vi "HS_DAQ_Host.vi"() -> ()   [LabVIEW 2020]
panel:
  out "Temperature [°C]":dbl format="%#_3g"
  out "Pulse count":dbl format="%#_3g"
  out "Frequency [Hz]":dbl format="%#_3g"
  out "Waveform Chart":dbl[][](graph)
  in  "Log data":bool
  in  "Sample rate [Hz]":dbl=20000.0
  in  "stop":bool
  out "data out":dbl[][](array[numeric]) format="%#_3g"
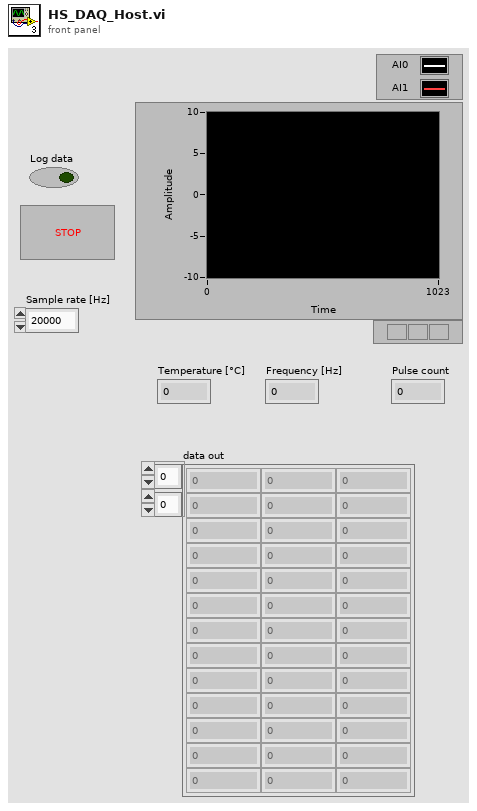
[diagram p1: front panel]
types:
  T1 = enum16{"open", "open or create", "create or replace", "create", "open (read-only)"}
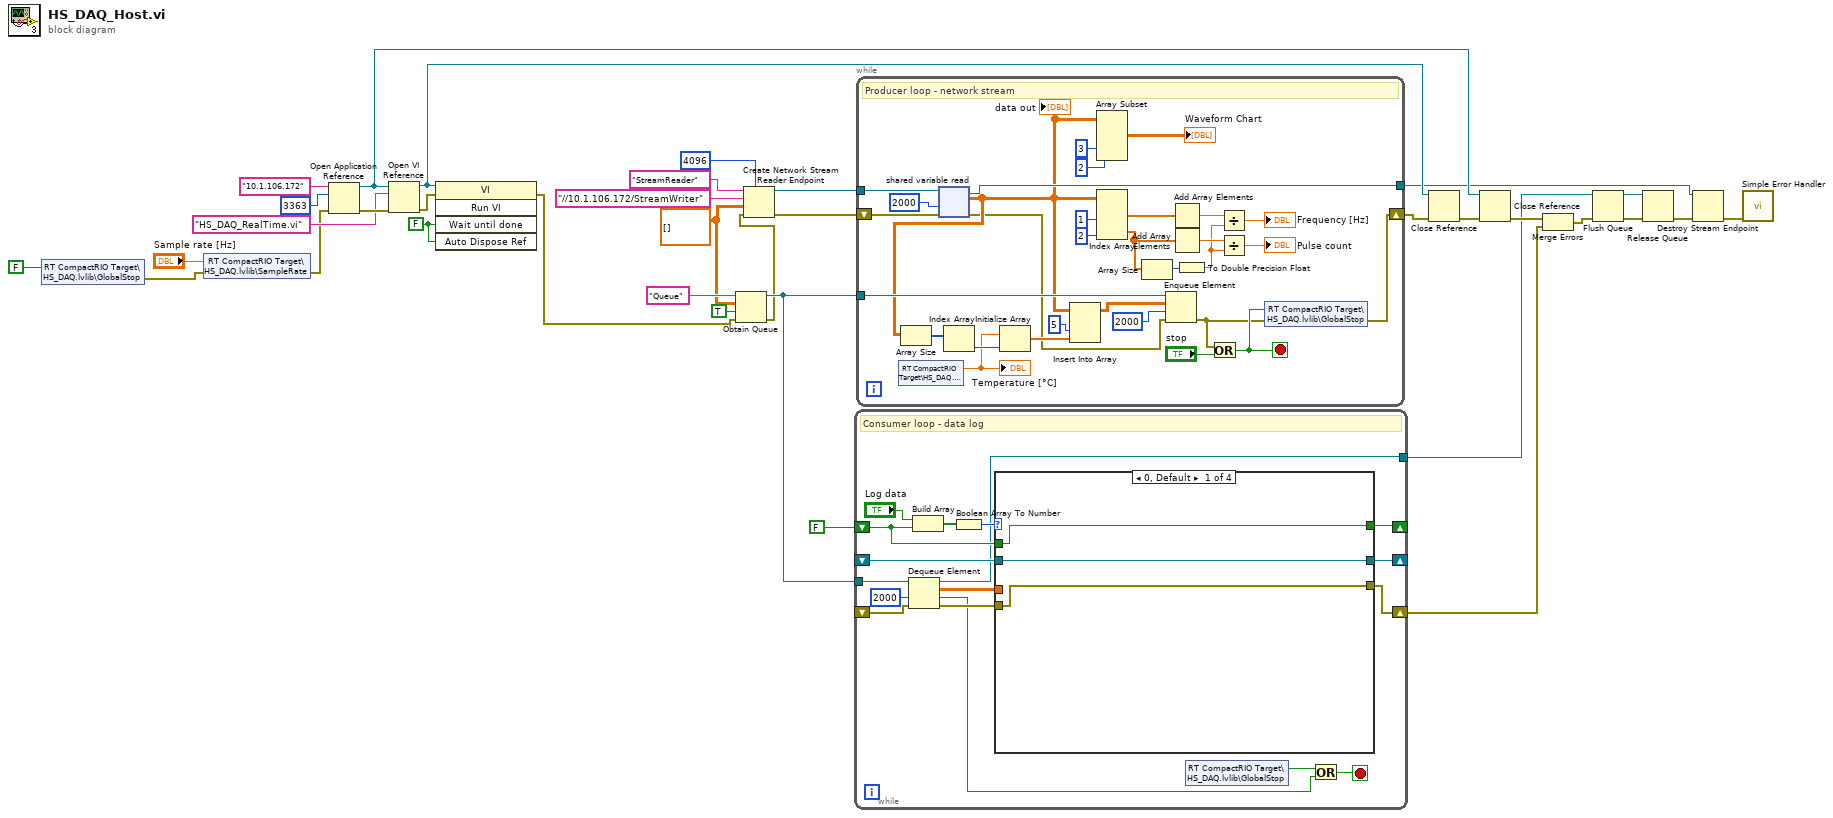
[diagram p0: block diagram]
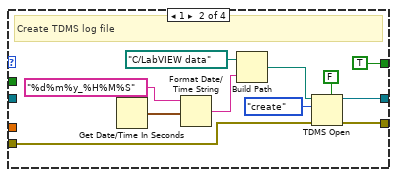
[diagram p2: hidden frame]
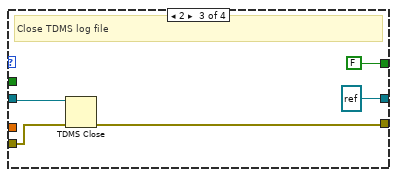
[diagram p3: hidden frame]
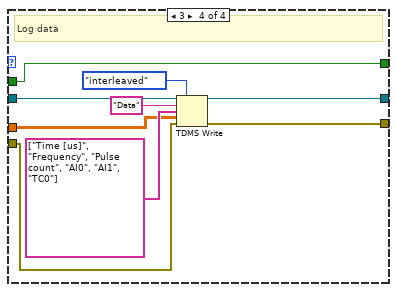
[diagram p4: hidden frame]
diagram:
  w26 = FALSE ("Wait Until Done")
  w24 = dbl[][] []
  n1 = shared-variable "RT CompactRIO Target\\HS_DAQ.lvlib\\GlobalStop"(FALSE ("GlobalStop")) -> (error out=w13:errorcluster)  [unwired: 1 in]
  n2 = shared-variable "RT CompactRIO Target\\HS_DAQ.lvlib\\SampleRate"("Sample rate [Hz]", error in=w13) -> (error out=w12:errorcluster)
  n3 = Open Application Reference(8:w12, 10:u16 3363 ("port number or service name (3363)"), 11:"10.1.106.172" ("machine name (\"\":  open local reference)")) -> (0:w29:errorcluster, 3:w19:refnum<vi>)  [unwired: 1 in]
  n4 = Open VI Reference(application reference (local)=w19, vi path="HS_DAQ_RealTime.vi" ("machine name (\"\":  open local reference)"), error in (no error)=w29) -> (vi reference=w20:refnum<vi>, error out=w27:errorcluster)  [unwired: 3 in]
  n5 = invoke class="VI" method="Run VI"(reference=w20, error in=w27, "Wait until done"=w26, "Auto Dispose Ref"=w26) -> (error out=w8:errorcluster)  [unwired: 1 in, 4 out]
  n6 = Obtain Queue(name (unnamed)="Queue", element data type=w24, create if not found? (T)=TRUE, error in (no error)=w8) -> (queue out=w23:refnum<queue>, error out=w7:errorcluster)  [unwired: 1 in, 1 out]
  n7 = Create Network Stream Reader Endpoint(7:4096 ("reader buffer size"), 8:w7, 9:w24, 10:"//10.1.106.172/StreamWriter" ("writer url"), 11:"StreamReader" ("reader name")) -> (0:w6:errorcluster, 3:w32:refnum<k21>)  [unwired: 2 in]
  n8 = while {
    tunnel: w23 -> [w52]
    shift-right: [w47] -> _
    shift-left: _ -> [w45]
    shift-right: [w46] -> _
    shift-left: FALSE -> [w44]
    shift-right: [w40] -> w3
    shift-left: _ -> [w42]
    tunnel: [w39] -> w1
    stop <- w38 stop-if-true
    # "Consumer loop - data log"
    n9 = Dequeue Element(queue=w52, timeout in ms (-1)=2000, error in (no error)=w42) -> (queue out=w39:refnum<queue>, element=w43:dbl[][], timed out?=w36:bool, error out=w41:errorcluster)
    n10 = Build Array("Log data", w44) -> (w48:bool[])
    n11 = Boolean Array To Number(Boolean array=w48) -> (number=w50:u32)
    n12 = case shown="0, Default" w50 {
      tunnel: [w55 w59 refnum<k34> refnum ("tdms file out") w75] -> w47
      tunnel: [w54 TRUE FALSE w74] -> w46
      tunnel: w45 -> [w55 _ w71 w80]
      tunnel: w44 -> [w54 _ _ w74]
      tunnel: w43 -> [_ _ _ w77]
      tunnel: w41 -> [w53 w57 w68 w73]
      tunnel: [w53 w56 w67 w72] -> w40
      frame 0, Default {
      }
      frame 1 {
        # "Create TDMS log file"
        n13 = Get Date/Time In Seconds() -> (seconds since 1Jan1904=w64:timestamp)
        n14 = Format Date/Time String(time format string (%c)="%d%m%y_%H%M%S", seconds (now)=w64) -> (date/time string=w62:string)  [unwired: 1 in]
        n15 = Build Path(base path=path "C:/LabVIEW data", name or relative path=w62) -> (appended path=w61:path)
        n16 = TDMS Open(5:FALSE ("create index file? (T)"), 8:w57, 10:T1."create" ("operation (0:open)"), 11:w61) -> (0:w56:errorcluster, 3:w59:refnum<k34>)  [unwired: 3 in]
      }
      frame 2 {
        # "Close TDMS log file"
        n17 = TDMS Close(8:w68, 11:w71) -> (0:w67:errorcluster)  [unwired: 1 out]
      }
      frame 3 {
        # "Log data"
        n18 = TDMS Write(0:w80, 1:enum16{"decimated", "interleaved"}."interleaved" ("data layout (0:decimated)"), 5:"Data" ("group name in (Untitled)"), 7:string[] ["Time [us]", "Frequency", "Pulse count", "AI0", "AI1", "TC0"] ("channel name(s) in (Untitled)"), 9:w77, 11:w73) -> (4:w75:refnum<k34>, 15:w72:errorcluster)  [unwired: 2 out]
      }
    }
    n19 = shared-variable "RT CompactRIO Target\\HS_DAQ.lvlib\\GlobalStop"() -> (w37:bool)  [unwired: 1 in, 1 out]
    n20 = Or(x=w37, y=w36) -> (x .or. y?=w38:bool)
  }
  n21 = while {
    tunnel: w32 -> [w111]
    shift-right: [w102] -> w11
    shift-left: w6 -> [w110]
    tunnel: w23 -> [w106]
    tunnel: [w104] -> w9
    stop <- w108 stop-if-true
    # "Producer loop - network stream"
    n22 = shared-variable "RT CompactRIO Target\\HS_DAQ.lvlib\\TC0"() -> (w85:dbl)  [unwired: 1 in, 1 out]
    "Temperature [°C]" <- w85
    n23 = shared-variable-read(w111, w110, 2000 ("timeout ms (-1)")) -> (w104:refnum<k21>, w82:errorcluster, w88:dbl[][])  [unwired: 1 out]
    "data out" <- w88
    n24 = Array Size(array=w88) -> (size(s)=w87:i32[])
    n25 = Index Array(array=w87) -> (element=w86:i32)  [unwired: 1 in]
    n26 = Initialize Array(w85, w86) -> (w84:dbl[])
    n27 = Insert Into Array(array=w88, index (col)=5 ("disabled index (col)"), new element=w84) -> (w83:dbl[][])  [unwired: 1 in]
    n28 = Array Subset(array=w88, index (col)=3 ("index"), length (col)=2 ("length")) -> (→"Waveform Chart":dbl[][])  [unwired: 2 in]
    n29 = Index Array(array=w88, index (col) #1=1 ("disabled index (col)"), index (col) #2=2 ("index (col)")) -> (element #1=w96:dbl[], element #2=w93:dbl[])  [unwired: 2 in]
    n30 = Array Size(array=w93) -> (size(s)=w92:i32)
    n31 = Enqueue Element(queue=w106, element=w83, timeout in ms (-1)=2000, error in (no error)=w82) -> (error out=w103:errorcluster)  [unwired: 2 out]
    n32 = Add Array Elements(numeric array=w96) -> (sum=w95:dbl)
    n33 = Add Array Elements(numeric array=w93) -> (sum=w94:dbl)
    n34 = To Double Precision Float(number=w92) -> (double precision float=w89:dbl)
    n35 = Or(x=w103, y="stop") -> (x .or. y?=w108:bool)
    n36 = Divide(x=w95, y=w89) -> (x/y=→"Frequency [Hz]":dbl)
    n37 = Divide(x=w94, y=w89) -> (x/y=→"Pulse count":dbl)
    n38 = shared-variable "RT CompactRIO Target\\HS_DAQ.lvlib\\GlobalStop"(w108, error in=w103) -> (error out=w102:errorcluster)
  }
  n39 = Close Reference(reference=w20, error in (no error)=w11) -> (error out=w21:errorcluster)
  n40 = Close Reference(reference=w19, error in (no error)=w21) -> (error out=w5:errorcluster)
  n41 = Merge Errors(w5, w3) -> (w4:errorcluster)
  n42 = Flush Queue(queue=w1, error in (no error)=w4) -> (queue out=w17:refnum<queue>, error out=w16:errorcluster)  [unwired: 1 out]
  n43 = Release Queue(queue=w17, error in (no error)=w16) -> (error out=w10:errorcluster)  [unwired: 1 in, 2 out]
  n44 = Destroy Stream Endpoint(8:w10, 11:w9) -> (0:w2:errorcluster)
  n45 = call <vilib>:"Simple Error Handler.vi"("error in (no error)"=w2) -> ()  [unwired: 4 in, 5 out]
